vi "MdfStart.vi"(8 "error in (no error)":errorcluster, 9 "start_time":u64, 11 "MDFRef":refnum<k24>) -> (0 "error IO":errorcluster, 1 "InitMeasurement":bool, 3 "MDFRef out":refnum<k24>)   [LabVIEW 2025, in "MdfFile.lvlib"]
uses:
  MdfFile.lvlib
  data/mdflibrary.dll
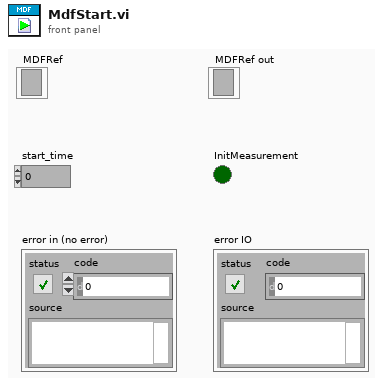
[diagram p1: front panel]
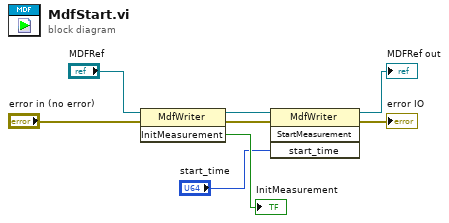
[diagram p0: block diagram]
diagram:
  n1 = invoke class="MdfWriter" method="InitMeasurement"(reference="MDFRef", error in="error in (no error)") -> (reference out=w6:refnum<k24>, error out=w4:errorcluster, "InitMeasurement"=→"InitMeasurement":bool)  [unwired: 1 in]
  n2 = invoke class="MdfWriter" method="StartMeasurement"(reference=w6, error in=w4, "start_time"="start_time") -> (reference out=→"MDFRef out":refnum<k24>, error out=→"error IO":errorcluster)  [unwired: 1 in, 2 out]
